vi "img_update_frame_count.vi"(8 "error in":errorcluster, 9 "sector size (512)":u32=512, 10 "Frame Count":u32, 11 "hFile":i64) -> (0 "error out":errorcluster, 3 "hFile":i64)   [LabVIEW 2016]
uses:
  kernel32.dll
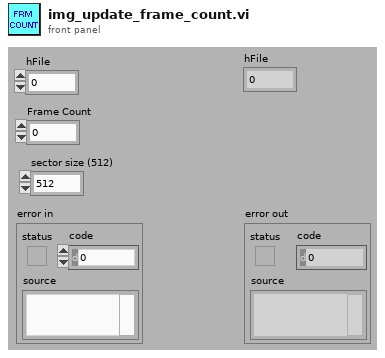
[diagram p1: front panel]
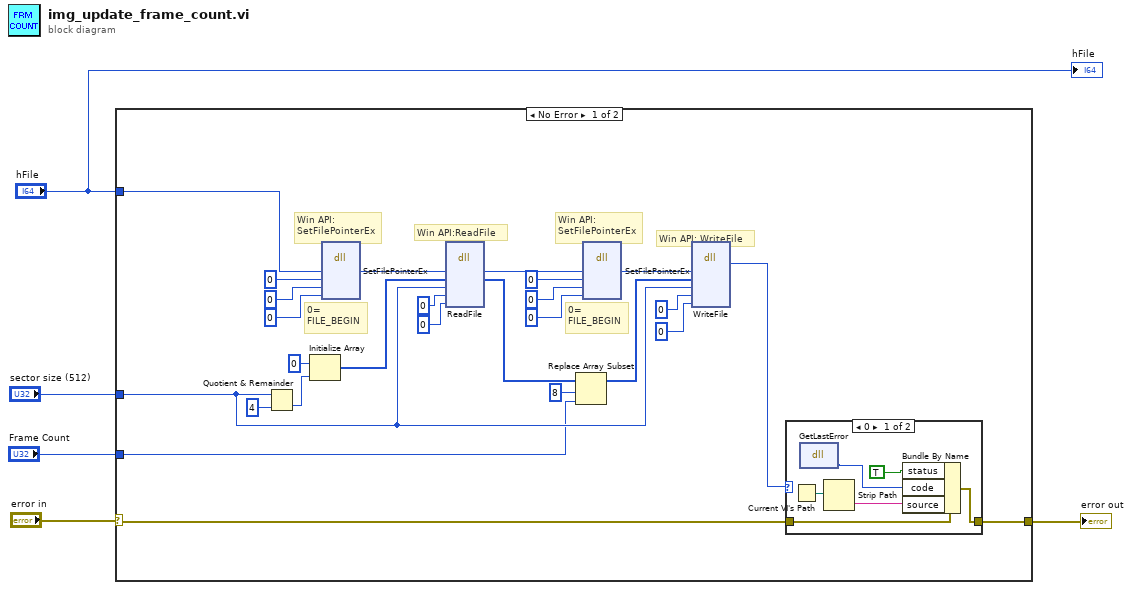
[diagram p0: block diagram]
diagram:
  n1 = case shown="No Error" "error in" {
    selector: "error in" -> [w31 w39]
    tunnel: "hFile" -> [w29 _]
    tunnel: [w30 w39] -> w5
    tunnel: "sector size (512)" -> [w28 _]
    tunnel: "Frame Count" -> [w27 _]
    frame No Error {
      # "Win API: WriteFile"
      # "Win API:\nSetFilePointerEx"
      # "0=\nFILE_BEGIN"
      # "Win API:\nSetFilePointerEx"
      # "0=\nFILE_BEGIN"
      # "Win API:ReadFile"
      n2 = Quotient & Remainder(x=w28, y=u32 4 ("element")) -> (floor(x/y)=w19:u32)  [unwired: 1 out]
      n3 = Initialize Array(u32 0 ("element"), w19) -> (w18:u32[])
      n4 = dll-call lib="kernel32.dll" fn="SetFilePointerEx"("hFile"=w29, "lDistanceToMove"=i64 0 ("lpNewFilePointer"), "lpNewFilePointer"=i64 0, "dwMoveMethod"=u32 0) -> ("hFile"=w17:i64)  [unwired: 5 in, 4 out]
      n5 = dll-call lib="kernel32.dll" fn="ReadFile"("hFile"=w17, "lpBuffer"=w18, "nNumberOfBytesToRead"=w28, "lpNumberOfBytesRead"=u32 0 ("lpOverlapped"), "lpOverlapped"=u32 0) -> ("hFile"=w12:i64, "lpBuffer"=w16:u32[])  [unwired: 5 in, 4 out]
      n6 = Replace Array Subset(array=w16, new element=w27, index=8) -> (w8:u32[])
      n7 = dll-call lib="kernel32.dll" fn="SetFilePointerEx"("hFile"=w12, "lDistanceToMove"=i64 0 ("lpNewFilePointer"), "lpNewFilePointer"=i64 0, "dwMoveMethod"=u32 0) -> ("hFile"=w9:i64)  [unwired: 5 in, 4 out]
      n8 = dll-call lib="kernel32.dll" fn="WriteFile"("hFile"=w9, "lpBuffer"=w8, "nNumberOfBytesToWrite"=w28, "lpNumberOfBytesWritten"=u32 0, "lpOverlapped"=u32 0) -> ("error"=w6:i32)  [unwired: 7 in, 3 out]
      n9 = case shown="0" w6 {
        tunnel: w31 -> [w37 w38]
        tunnel: [w36 w38] -> w30
        frame 0 {
          n10 = Current VI's Path() -> (path=w34:path)
          n11 = dll-call lib="kernel32.dll" fn="GetLastError"() -> ("error"=w32:u32)  [unwired: 3 in, 2 out]
          n12 = Strip Path(path=w34) -> (name=w33:string)  [unwired: 1 out]
          n13 = Bundle By Name(cluster=w37, "status"=TRUE, "code"=w32, "source"=w33) -> (w36:errorcluster)
        }
        frame 1, Default {
        }
      }
    }
    frame Error {
    }
  }
  "error out" <- w5
  "hFile" <- "hFile"
